vi "Begin.vi"() -> (0 "error out":errorcluster)   [LabVIEW 2018]
doc: "Called before other user functions, this VI can be used to open I/O refnums, load in file data, and do general program initialization. Notice that the <B>error out</B> terminal is simply used for data flow. Wiring it to other structures or subVIs ensures that this VI runs first."
uses:
  <vilib>/Rock Robotics/WPI/DriverStation/WPI_DriverStationRobotMode2.ctl
  <vilib>/Rock Robotics/WPI/Joystick/WPI_JoystickDeviceEnum.ctl
  <vilib>/Rock Robotics/WPI/ThirdParty/REV Robotics/SPARK MAX/Typedef/Spark MAX Status Frames.ctl
  <vilib>/Rock Robotics/WPI/Solenoid/WPI_SolenoidChannel.ctl
  <vilib>/Rock Robotics/WPI/ThirdParty/REV Robotics/SPARK MAX/Typedef/Spark MAX Motor Type.ctl
  <vilib>/Rock Robotics/SystemInterfaces/DIO/FPGA_DIOChannel.ctl
  <vilib>/Rock Robotics/WPI/ThirdParty/REV Robotics/SPARK MAX/Typedef/Spark MAX Idle Mode.ctl
  <vilib>/Rock Robotics/WPI/Solenoid/WPI_SolenoidValue.ctl
  <vilib>/Rock Robotics/WPI/SafetyOutput/WPI_SafetyOutputConfigMenu.ctl
  Odometry/Typedef/Odometry.ctl
  Robot Global Data.vi
  <vilib>/Rock Robotics/Network Tables/NT Write String Array.vi
  <vilib>/Rock Robotics/WPI/Solenoid/WPI_SolenoidOpenDouble.vi
  <vilib>/Rock Robotics/WPI/Counter/WPI_CounterDigitalInputToDigitalSource.vi
  <vilib>/Rock Robotics/WPI/Counter/WPI_CounterOpen Semi Period Mode.vi
  <vilib>/Rock Robotics/WPI/Solenoid/WPI_SolenoidSetEnum.vi
  Asynchronous TDMS Logger/TDMS Logger.lvclass
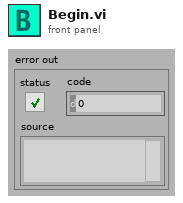
[diagram p1: front panel]
types:
  T1 = typedef "WPI_SafetyOutputConfigMenu.ctl" = enum16{"Enable", "Disable"}
  T2 = typedef "WPI_SolenoidValue.ctl" = enum16{"Off", "On", "Forward", "Reverse"}
  T3 = typedef "WPI_SolenoidChannel.ctl" = enum8{"Solenoid 0", "Solenoid 1", "Solenoid 2", "Solenoid 3", "Solenoid 4", "Solenoid 5", "Solenoid 6", "Solenoid 7", "Invalid"}
  T4 = typedef "FPGA_DIOChannel.ctl" = enum8{"DIO 0", "DIO 1", "DIO 2", "DIO 3", "DIO 4", "DIO 5", "DIO 6", "DIO 7", "DIO 8", "DIO 9", "DIO MXP 0", "DIO MXP 1", "DIO MXP 2", "DIO MXP 3", "DIO MXP 4", "DIO MXP 5", "DIO MXP 6", "DIO MXP 7", "DIO MXP 8", "DIO MXP 9", "DIO MXP 10", "DIO MXP 11", "DIO MXP 12", "DIO MXP 13", "DIO MXP 14", "DIO MXP 15", "SPI Port CS1", "SPI Port CS2", "SPI Port CS3", "SPI Port MISO", "SPI Port MOSI", "Invalid"}
  T5 = typedef "Spark MAX Status Frames.ctl" = enum16{"Status 0", "Status 1", "Status 2"}
  T6 = typedef "Spark MAX Idle Mode.ctl" = enum16{"Coast", "Brake"}
  T7 = typedef "Spark MAX Motor Type.ctl" = enum16{"Brushed", "Brushless"}
  T8 = cluster{"P Gain":dbl, "I Gain":dbl, "D Gain":dbl, "F Gain":dbl, "I Zone":dbl, "Min Output":dbl, "Max Output":dbl}
  T9 = typedef "WPI_JoystickDeviceEnum.ctl" = enum16{"USB 0", "USB 1", "USB 2", "USB 3", "USB 4", "USB 5"}
  T10 = typedef "WPI_DriverStationRobotMode2.ctl" = enum16{"Autonomous Disabled", "Autonomous Enabled", "Teleop Disabled", "Teleop Enabled", "Disconnected", "Finish", "Test Disabled", "Test Enabled", "Emergency Stopped"}
  T11 = typedef "WPI_MotorControlDeviceRef.ctl" = cluster{"DeviceStatus":errorcluster, "Type":T12, "PWM":cluster{"PWM Channel":T13, "DeadBand":T14}, "CAN":cluster{"Device Number":u8, "SetOutput VI Ref":variant, "GetOutput VI Ref":variant, "Enable VI Ref":variant, "Disable VI Ref":variant, "Data":variant}, "Invert":bool, "DIO PWM":cluster{"PWM \"Enable\" Channel":T13, "DIOChannel":T4, "PWM Rate":dbl}}
  T12 = typedef "WPI_MotorControlType.ctl" = enum16{"PWM", "CAN", "DIO PWM"}
  T13 = typedef "FPGA_DIOPWMChannel.ctl" = enum8{"PWM 0", "PWM 1", "PWM 2", "PWM 3", "PWM 4", "PWM 5", "PWM 6", "PWM 7", "PWM 8", "PWM 9", "PWM MXP 0", "PWM MXP 1", "PWM MXP 2", "PWM MXP 3", "PWM MXP 4", "PWM MXP 5", "PWM MXP 6", "PWM MXP 7", "PWM MXP 8", "PWM MXP 9", "Invalid"}
  T14 = typedef "WPI_PWMDeadband.ctl" = cluster{"Name":string, "maxPositivePwm":i32, "minPositivePwm":i32, "centerPwm":i32, "maxNegativePwm":i32, "minNegativePwm":i32, "angularRange":u16}
  T15 = typedef "WPI_DigitalInputDevRef.ctl" = cluster{"DevStatus":errorcluster, "DIO Channel":T4}
  T16 = typedef "FPGA_CounterEncoderSourceConvertionLVSourceType.ctl" = cluster{"DevStatus":errorcluster, "AnalogTriggerMode?":bool, "DigitalMode":cluster{"DIO Channel":T17}, "AnalogTriggerMode":cluster{"AnalogTriggerIndex":T18, "OutputType":T19}}
  T17 = typedef "FPGA_DIODigitalSourceChannel.ctl" = enum8{"DIO 0", "DIO 1", "DIO 2", "DIO 3", "DIO 4", "DIO 5", "DIO 6", "DIO 7", "DIO 8", "DIO 9", "DIO MXP 0", "DIO MXP 1", "DIO MXP 2", "DIO MXP 3", "DIO MXP 4", "DIO MXP 5", "DIO MXP 6", "DIO MXP 7", "DIO MXP 8", "DIO MXP 9", "DIO MXP 10", "DIO MXP 11", "DIO MXP 12", "DIO MXP 13", "DIO MXP 14", "DIO MXP 15", "SPI Port CS1", "SPI Port CS2", "SPI Port CS3", "SPI Port MISO", "SPI Port MOSI", "Disabled"}
  T18 = typedef "FPGA_AnalogTriggerIndex.ctl" = enum8{"Trig 0", "Trig 1", "Trig 2", "Trig 3", "Trig 4", "Trig 5", "Trig 6", "Trig 7", "Invalid"}
  T19 = typedef "FPGA_AnalogTriggerOutType.ctl" = enum16{"InWindow", "TriggerState", "Rising", "Falling"}
  T20 = typedef "WPI_EncoderDevRef.ctl" = cluster{"DevStatus":errorcluster, "EncoderIndex":T21, "CounterIndex":T22, "DistancePerCount":dbl, "Decoding Type":T23}
  T21 = typedef "FPGA_EncoderIdx.ctl" = enum8{"Enc 0", "Enc 1", "Enc 2", "Enc 3", "Enc 4", "Enc 5", "Enc 6", "Enc 7", "Invalid"}
  T22 = typedef "FPGA_CounterCtrSystemIndex.ctl" = enum8{"Ctr 0", "Ctr 1", "Ctr 2", "Ctr 3", "Ctr 4", "Ctr 5", "Ctr 6", "Ctr 7", "Invalid"}
  T23 = typedef "WPI_EncoderType.ctl" = enum16{"1x", "2x", "4x"}
  T24 = typedef "WPI_JoystickDevRef.ctl" = cluster{"Device":T9}
  T25 = typedef "Odometry.ctl" = cluster{"x":dbl, "y":dbl, "theta":dbl, "Left Encoder":dbl, "Right Encoder":dbl, "Late Iterations":i16}
  T26 = typedef "SPARKMAX6Motor.ctl" = cluster{"FrontLeftMaster":T11, "FrontLeftSlave1":T11, "FrontLeftSlave2":T11, "FrontRightMaster":T11, "FrontRightSlave1":T11, "FrontRightSlave2":T11}
  T27 = typedef "WPI_SolenoidDevRef.ctl" = cluster{"DevStatus":errorcluster, "Pneumatics Control Module":u8, "Forward Solenoid Channel":T3, "Reverse Solenoid Channel":T3}
  T28 = typedef "WPI_CounterDevRef.ctl" = cluster{"DevStatus":errorcluster, "CntIndex":T22}
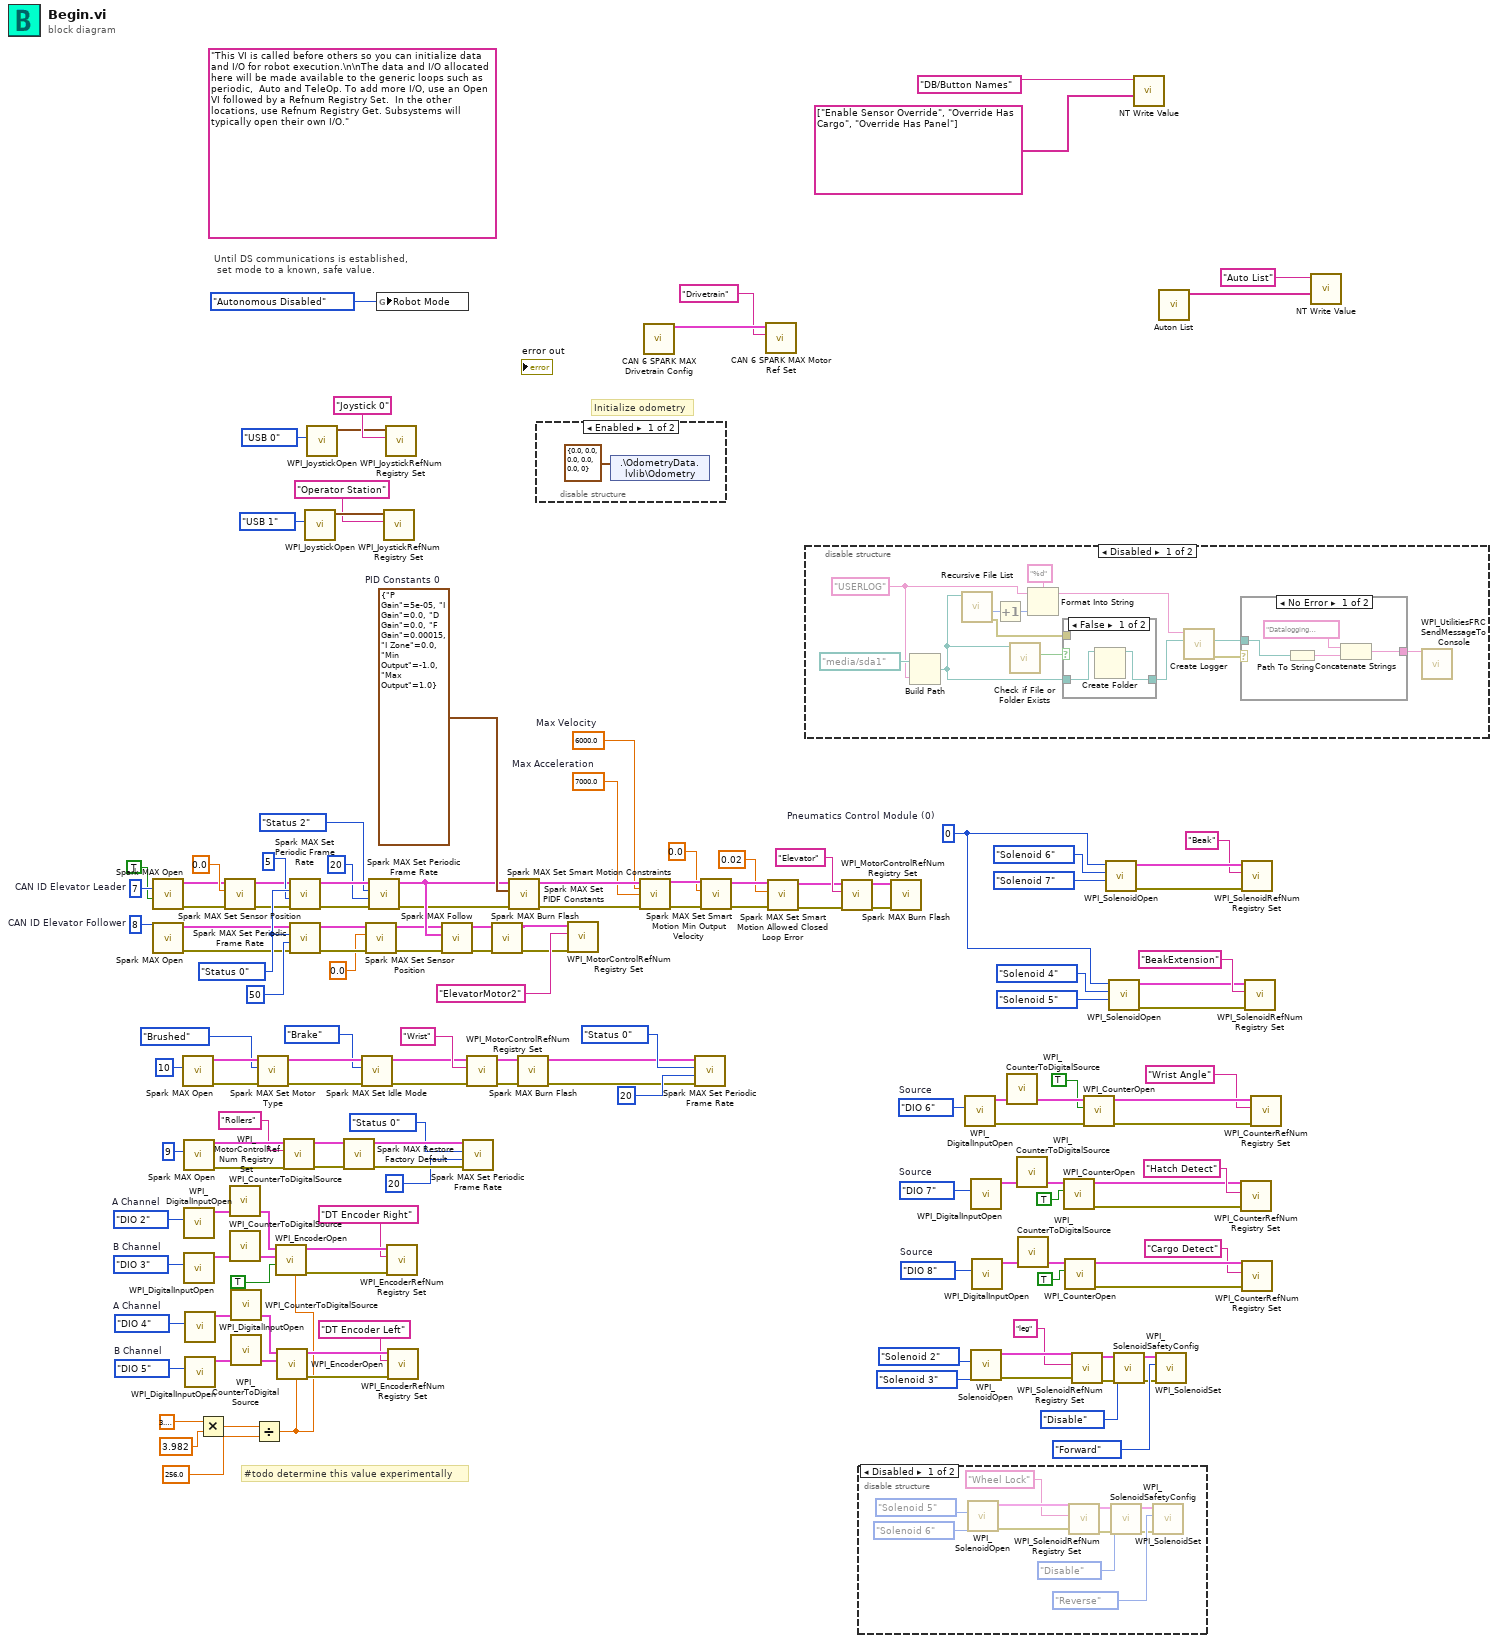
[diagram p0: block diagram]
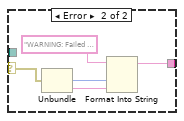
[diagram p5: hidden frame]
diagram:
  w14 = FPGA_DIOChannel."DIO 8"  # Source
  w39 = FPGA_DIOChannel."DIO 5"  # B Channel
  w40 = FPGA_DIOChannel."DIO 4"  # A Channel
  w50 = FPGA_DIOChannel."DIO 3"  # B Channel
  w49 = FPGA_DIOChannel."DIO 2"  # A Channel
  w64 = FPGA_DIOChannel."DIO 7"  # Source
  w80 = 7000.0  # Max Acceleration
  w81 = 6000.0  # Max Velocity
  w94 = FPGA_DIOChannel."DIO 6"  # Source
  w107 = u8 0  # Pneumatics Control Module (0)
  w138 = T8 {"P Gain"=5e-05, "I Gain"=0.0, "D Gain"=0.0, "F Gain"=0.00015, "I Zone"=0.0, "Min Output"=-1.0, "Max Output"=1.0}  # PID Constants 0
  w136 = Spark_MAX_Status_Frames."Status 0" ("Frame")
  w132 = u8 7  # CAN ID Elevator Leader
  w133 = u8 8  # CAN ID Elevator Follower
  (unwired) "This VI is called before others so you can initialize data and I/O for robot execution.\n\nThe data and I/O allocated here will be made available to the generic loops such as periodic,  Auto and TeleOp. To add more I/O, use an Open VI followed by a Refnum Registry Set.  In the other locations, use Refnum Registry Get. Subsystems will typically open their own I/O."
  # "#todo determine this value experimentally"
  # "Initialize odometry"
  # "Until DS communications is established,\n set mode to a known, safe value."
  n1 = call <vilib>:"Spark MAX Open.vi"("Invert"=TRUE, "Device Number"=w132) -> ("error out"=w122:errorcluster, "MotorControlDeviceRef"=w121:T11)  [unwired: 8 in]
  n2 = call <vilib>:"Spark MAX Open.vi"("Device Number"=w133) -> ("error out"=w134:errorcluster, "MotorControlDeviceRef"=w135:T11)  [unwired: 9 in]
  n3 = call <vilib>:"Spark MAX Open.vi"("Device Number"=u8 10) -> ("error out"=w75:errorcluster, "MotorControlDeviceRef"=w99:T11)  [unwired: 9 in]
  n4 = call <vilib>:"Spark MAX Open.vi"("Device Number"=u8 9) -> ("error out"=w68:errorcluster, "MotorControlDeviceRef"=w101:T11)  [unwired: 9 in]
  n5 = call <vilib>:"WPI_DigitalInputOpen.vi"("DIO Channel"=w49) -> ("DigitalInputDevRef"=w46:T15)  [unwired: 1 in, 9 out]
  n6 = call <vilib>:"WPI_DigitalInputOpen.vi"("DIO Channel"=w50) -> ("DigitalInputDevRef"=w47:T15)  [unwired: 1 in, 9 out]
  n7 = call <vilib>:"WPI_DigitalInputOpen.vi"("DIO Channel"=w40) -> ("DigitalInputDevRef"=w43:T15)  [unwired: 1 in, 9 out]
  n8 = call <vilib>:"WPI_DigitalInputOpen.vi"("DIO Channel"=w39) -> ("DigitalInputDevRef"=w42:T15)  [unwired: 1 in, 9 out]
  n9 = Multiply(x=3.141592653589793, y=3.982) -> (x*y=w30:dbl)
  n10 = call <vilib>:"Spark MAX Set Sensor Position.vi"("error in"=w122, "Position"=0.0, "MotorControlDeviceRef"=w121) -> ("error out"=w119:errorcluster, "MotorControlDeviceRef"=w120:T11)  [unwired: 7 in]
  n11 = call-poly <vilib>:"WPI_CounterToDigitalSource.vi"("DigitalInputDevRef"=w46) -> ("Digital Source"=w45:T16)  [unwired: 6 out]
  n12 = call-poly <vilib>:"WPI_CounterToDigitalSource.vi"("DigitalInputDevRef"=w47) -> ("Digital Source"=w48:T16)  [unwired: 6 out]
  n13 = call-poly <vilib>:"WPI_CounterToDigitalSource.vi"("DigitalInputDevRef"=w43) -> ("Digital Source"=w44:T16)  [unwired: 6 out]
  n14 = call-poly <vilib>:"WPI_CounterToDigitalSource.vi"("DigitalInputDevRef"=w42) -> ("Digital Source"=w41:T16)  [unwired: 6 out]
  n15 = Divide(x=w30, y=256.0) -> (x/y=w1:dbl)
  n16 = call <vilib>:"Spark MAX Set Motor Type.vi"("error in (no error)"=w75, "Enum"=Spark_MAX_Motor_Type."Brushed", "MotorControlDevRef"=w99) -> ("error out"=w96:errorcluster, "MotorControlDeviceRef"=w73:T11)  [unwired: 7 in]
  n17 = call <vilib>:"WPI_EncoderOpen.vi"("DistancePerCount"=w1, "Invert Direction (False)"=TRUE, "BSource"=w48, "ASource"=w45) -> ("error out"=w38:errorcluster, "EncoderDevRef"=w35:T20)  [unwired: 4 in, 2 out]
  n18 = call <vilib>:"WPI_EncoderOpen.vi"("DistancePerCount"=w1, "BSource"=w41, "ASource"=w44) -> ("error out"=w37:errorcluster, "EncoderDevRef"=w36:T20)  [unwired: 5 in, 2 out]
  n19 = call <vilib>:"WPI_MotorControlRefNum Registry Set.vi"("error in (no error)"=w68, "refnum name"="Rollers", "MotorControlDevRef"=w101) -> ("error out"=w67:errorcluster, "MotorControlDevRef"=w66:T11)  [unwired: 7 in]
  n20 = call <vilib>:"Spark MAX Set Periodic Frame Rate.vi"("error in"=w119, "Frame rate (ms)"=u16 5, "Frame"=w136, "MotorControlDeviceRef"=w120) -> ("error out"=w131:errorcluster, "MotorControlDeviceRef"=w130:T11)  [unwired: 6 in]
  n21 = call <vilib>:"Spark MAX Set Periodic Frame Rate.vi"("error in"=w134, "Frame rate (ms)"=u16 50, "Frame"=w136, "MotorControlDeviceRef"=w135) -> ("error out"=w54:errorcluster, "MotorControlDeviceRef"=w55:T11)  [unwired: 6 in]
  n22 = call <vilib>:"WPI_JoystickOpen.vi"("JoystickDevice"=WPI_JoystickDeviceEnum."USB 1") -> ("JoystickDevRef"=w145:T24)  [unwired: 10 in]
  n23 = call <vilib>:"WPI_JoystickOpen.vi"("JoystickDevice"=WPI_JoystickDeviceEnum."USB 0") -> ("JoystickDevRef"=w150:T24)  [unwired: 10 in]
  n24 = call <vilib>:"Spark MAX Restore Factory Default.vi"("error in"=w67, "MotorControlDeviceRef"=w66) -> ("error out"=w26:errorcluster, "MotorControlDeviceRef"=w27:T11)  [unwired: 8 in]
  n25 = call <vilib>:"Spark MAX Set Idle Mode.vi"("error in (no error)"=w96, "Idle Mode"=Spark_MAX_Idle_Mode."Brake", "MotorControlDeviceRef in"=w73) -> ("error out"=w74:errorcluster, "MotorControlDeviceRef out"=w72:T11)  [unwired: 7 in]
  n26 = call <vilib>:"Spark MAX Set Sensor Position.vi"("error in"=w54, "Position"=0.0, "MotorControlDeviceRef"=w55) -> ("error out"=w52:errorcluster, "MotorControlDeviceRef"=w53:T11)  [unwired: 7 in]
  n27 = call <vilib>:"Spark MAX Set Periodic Frame Rate.vi"("error in"=w131, "Frame rate (ms)"=u16 20, "Frame"=Spark_MAX_Status_Frames."Status 2", "MotorControlDeviceRef"=w130) -> ("error out"=w127:errorcluster, "MotorControlDeviceRef"=w129:T11)  [unwired: 6 in]
  n28 = global write "Robot Global Data.vi" "Robot Mode"(WPI_DriverStationRobotMode2."Autonomous Disabled" ("Robot Mode")) -> ()
  n29 = call <vilib>:"WPI_JoystickRefNum Registry Set.vi"("refnum name"="Operator Station", "JoystickDevRef"=w145) -> ()  [unwired: 8 in, 2 out]
  n30 = call <vilib>:"WPI_JoystickRefNum Registry Set.vi"("refnum name"="Joystick 0", "JoystickDevRef"=w150) -> ()  [unwired: 8 in, 2 out]
  n31 = call <vilib>:"WPI_EncoderRefNum Registry Set.vi"("error in (no error)"=w38, "refnum name"="DT Encoder Right", "EncoderDevRef"=w35) -> ()  [unwired: 7 in, 2 out]
  n32 = call <vilib>:"WPI_EncoderRefNum Registry Set.vi"("error in (no error)"=w37, "refnum name"="DT Encoder Left", "EncoderDevRef"=w36) -> ()  [unwired: 7 in, 2 out]
  n33 = call <vilib>:"Spark MAX Follow.vi"("error in (no error)"=w52, "Master Controller"=w129, "MotorControlDeviceRef"=w53) -> ("error out"=w105:errorcluster, "MotorControlDeviceRef"=w104:T11)  [unwired: 7 in]
  n34 = call <vilib>:"Spark MAX Set Periodic Frame Rate.vi"("error in"=w26, "Frame rate (ms)"=u16 20, "Frame"=Spark_MAX_Status_Frames."Status 0", "MotorControlDeviceRef"=w27) -> ()  [unwired: 6 in, 2 out]
  n35 = call <vilib>:"WPI_MotorControlRefNum Registry Set.vi"("error in (no error)"=w74, "refnum name"="Wrist", "MotorControlDevRef"=w72) -> ("error out"=w70:errorcluster, "MotorControlDevRef"=w69:T11)  [unwired: 7 in]
  n36 = call <vilib>:"Spark MAX Burn Flash.vi"("error in"=w105, "MotorControlDeviceRef"=w104) -> ("error out"=w57:errorcluster, "MotorControlDeviceRef"=w56:T11)  [unwired: 8 in]
  n37 = call <vilib>:"Spark MAX Set PIDF Constants.vi"("error in"=w127, "PID Constants"=w138, "MotorControlDeviceRef"=w129) -> ("error out"=w125:errorcluster, "MotorControlDeviceRef"=w124:T11)  [unwired: 7 in]
  n38 = call <vilib>:"Spark MAX Burn Flash.vi"("error in"=w70, "MotorControlDeviceRef"=w69) -> ("error out"=w20:errorcluster, "MotorControlDeviceRef"=w21:T11)  [unwired: 8 in]
  n39 = disable-structure shown="Enabled" {
    frame Enabled {
      n40 = shared-variable ".\\OdometryData.lvlib\\Odometry"(T25 {"x"=0.0, "y"=0.0, "theta"=0.0, "Left Encoder"=0.0, "Right Encoder"=0.0, "Late Iterations"=0} ("Odometry")) -> ()  [unwired: 1 in, 1 out]
    }
    frame Disabled {
    }
  }
  n41 = call <vilib>:"WPI_MotorControlRefNum Registry Set.vi"("error in (no error)"=w57, "refnum name"="ElevatorMotor2", "MotorControlDevRef"=w56) -> ()  [unwired: 7 in, 2 out]
  n42 = call <vilib>:"Spark MAX Set Smart Motion Constraints.vi"("MotorControlDeviceRef"=w124, "Max Velocity"=w81, "Max Acceleration"=w80, "error in"=w125) -> ("MotorControlDeviceRef"=w86:T11, "error out"=w87:errorcluster)  [unwired: 10 in]
  n43 = call "CAN 6 SPARK MAX Drivetrain Config.vi"() -> ("SPARK MAX Ref"=w141:T26)  [unwired: 19 in]
  n44 = call <vilib>:"Spark MAX Set Periodic Frame Rate.vi"("error in"=w20, "Frame rate (ms)"=u16 20, "Frame"=Spark_MAX_Status_Frames."Status 0", "MotorControlDeviceRef"=w21) -> ()  [unwired: 6 in, 2 out]
  n45 = call <vilib>:"Spark MAX Set Smart Motion Min Output Velocity.vi"("error in"=w87, "Minimum Velocity Output"=0.0, "MotorControlDeviceRef"=w86) -> ("error out"=w85:errorcluster, "MotorControlDeviceRef"=w84:T11)  [unwired: 7 in]
  n46 = call "CAN 6 SPARK MAX Motor Ref Set.vi"("refnum name"="Drivetrain", "TalonSRX6MotorRef in"=w141) -> ()  [unwired: 8 in, 2 out]
  n47 = call <vilib>:"Spark MAX Set Smart Motion Allowed Closed Loop Error.vi"("error in"=w85, "Allowed Closed Loop Error"=0.02, "MotorControlDeviceRef"=w84) -> ("error out"=w83:errorcluster, "MotorControlDeviceRef"=w82:T11)  [unwired: 7 in]
  n48 = disable-structure shown="Disabled" {
    frame Disabled {
      w161 = "USERLOG" ("Base File Name")
      n49 = Build Path(base path=path "/media/sda1", name or relative path=w161) -> (appended path=w163:path)
      n50 = call <vilib>:"Recursive File List.vi"("Folder Path"=w163) -> ("error out"=w158:errorcluster, "Number of Files"=w162:i32)  [unwired: 6 in, 3 out]
      n51 = Increment(x=w162) -> (x+1=w160:i32)
      n52 = call <vilib>:"Check if File or Folder Exists.vi"("path"=w163) -> ("file or folder exists?"=w164:bool)  [unwired: 8 in, 2 out]
      n53 = Format Into String(format string="%d", initial string=w161, w160) -> (resulting string=w157:string)  [unwired: 1 in, 1 out]
      n54 = case shown="False" w164 {
        tunnel: w163 -> [w168 w169]
        tunnel: [w167 w169] -> w154
        tunnel: w158 -> [_ _]
        frame False {
          n55 = Create Folder(path (use dialog)=w168) -> (created path=w167:path)  [unwired: 2 in, 2 out]
        }
        frame True {
        }
      }
      n56 = call "Create Logger.vi"("Base Folder"=w154, "Base File Name"=w157) -> ("Error Out"=w155:errorcluster, "Final Path"=w156:path)  [unwired: 7 in, 1 out]
      n57 = case shown="No Error" w155 {
        selector: w155 -> [_ w177]
        tunnel: w156 -> [w173 _]
        tunnel: [w170 w174] -> w166
        frame No Error {
          n58 = Path To String(path=w173) -> (string=w172:string)
          n59 = Concatenate Strings("Datalogging Initialized to: " ("string"), w172) -> (w170:string)
        }
        frame Error {
          n60 = Unbundle(w177) -> ("code"=w176:i32, "source"=w175:string)  [unwired: 1 out]
          n61 = Format Into String(initial string="WARNING: Failed to initialize datalogger! " ("string"), w176, w175) -> (resulting string=w174:string)  [unwired: 2 in, 1 out]
        }
      }
      n62 = call <vilib>:"WPI_UtilitiesFRC SendMessageToConsole.vi"("Message"=w166) -> ()  [unwired: 14 in, 1 out]
    }
    frame Enabled {
    }
  }
  n63 = call <vilib>:"WPI_MotorControlRefNum Registry Set.vi"("error in (no error)"=w83, "refnum name"="Elevator", "MotorControlDevRef"=w82) -> ("error out"=w76:errorcluster, "MotorControlDevRef"=w77:T11)  [unwired: 7 in]
  n64 = disable-structure shown="Disabled" {
    frame Disabled {
      n65 = call-poly <vilib>:"WPI_SolenoidOpen.vi"("Reverse Solenoid Channel"=WPI_SolenoidChannel."Solenoid 6", "Forward Solenoid Channel"=WPI_SolenoidChannel."Solenoid 5" ("Solenoid Channel")) -> ("error out"=w187:errorcluster, "SolenoidDevRef"=w189:T27)  [unwired: 8 in]
      n66 = call <vilib>:"WPI_SolenoidRefNum Registry Set.vi"("error in (no error)"=w187, "refnum name"="Wheel Lock", "SolenoidDevRef"=w189) -> ("error out"=w182:errorcluster, "SolenoidDevRef"=w183:T27)  [unwired: 7 in]
      n67 = call <vilib>:"WPI_SolenoidSafetyConfig.vi"("error in (no error)"=w182, "mode"=WPI_SafetyOutputConfigMenu."Disable", "SolenoidDevRef"=w183) -> ("error out"=w180:errorcluster, "SolenoidDevRef"=w181:T27)  [unwired: 7 in]
      n68 = call-poly <vilib>:"WPI_SolenoidSet.vi"("error in (no error)"=w180, "Value"=WPI_SolenoidValue."Reverse", "SolenoidDevRef"=w181) -> ()  [unwired: 7 in, 2 out]
    }
    frame Enabled {
    }
  }
  n69 = call <vilib>:"Spark MAX Burn Flash.vi"("error in"=w76, "MotorControlDeviceRef"=w77) -> ()  [unwired: 8 in, 2 out]
  n70 = call <vilib>:"WPI_DigitalInputOpen.vi"("DIO Channel"=w94) -> ("error out"=w92:errorcluster, "DigitalInputDevRef"=w93:T15)  [unwired: 1 in, 8 out]
  n71 = call <vilib>:"WPI_DigitalInputOpen.vi"("DIO Channel"=w64) -> ("DigitalInputDevRef"=w63:T15)  [unwired: 1 in, 9 out]
  n72 = call-poly <vilib>:"WPI_SolenoidOpen.vi"("Reverse Solenoid Channel"=WPI_SolenoidChannel."Solenoid 3", "Forward Solenoid Channel"=WPI_SolenoidChannel."Solenoid 2" ("Solenoid Channel")) -> ("error out"=w10:errorcluster, "SolenoidDevRef"=w12:T27)  [unwired: 8 in]
  n73 = call <vilib>:"WPI_DigitalInputOpen.vi"("DIO Channel"=w14) -> ("DigitalInputDevRef"=w15:T15)  [unwired: 1 in, 9 out]
  n74 = call-poly <vilib>:"WPI_CounterToDigitalSource.vi"("DigitalInputDevRef"=w93) -> ("Digital Source"=w95:T16)  [unwired: 6 out]
  n75 = call-poly <vilib>:"WPI_CounterToDigitalSource.vi"("DigitalInputDevRef"=w63) -> ("Digital Source"=w65:T16)  [unwired: 6 out]
  n76 = call-poly <vilib>:"WPI_CounterToDigitalSource.vi"("DigitalInputDevRef"=w15) -> ("Digital Source"=w13:T16)  [unwired: 6 out]
  n77 = call-poly <vilib>:"WPI_CounterOpen.vi"("High Pulse (T)"=TRUE, "Source"=w65) -> ("error out"=w59:errorcluster, "CounterDevRef"=w60:T28)  [unwired: 3 in, 5 out]
  n78 = call-poly <vilib>:"WPI_CounterOpen.vi"("High Pulse (T)"=TRUE, "Source"=w13) -> ("error out"=w19:errorcluster, "CounterDevRef"=w18:T28)  [unwired: 3 in, 5 out]
  n79 = call <vilib>:"WPI_SolenoidRefNum Registry Set.vi"("error in (no error)"=w10, "refnum name"="leg", "SolenoidDevRef"=w12) -> ("error out"=w5:errorcluster, "SolenoidDevRef"=w6:T27)  [unwired: 7 in]
  n80 = call-poly <vilib>:"WPI_CounterOpen.vi"("error in (no error)"=w92, "High Pulse (T)"=TRUE, "Source"=w95) -> ("error out"=w90:errorcluster, "CounterDevRef"=w91:T28)  [unwired: 2 in, 5 out]
  n81 = call-poly <vilib>:"WPI_SolenoidOpen.vi"("Reverse Solenoid Channel"=WPI_SolenoidChannel."Solenoid 7", "Forward Solenoid Channel"=WPI_SolenoidChannel."Solenoid 6", "Pneumatics Control Module (0)"=w107) -> ("error out"=w116:errorcluster, "SolenoidDevRef"=w117:T27)  [unwired: 7 in]
  n82 = call-poly <vilib>:"WPI_SolenoidOpen.vi"("Reverse Solenoid Channel"=WPI_SolenoidChannel."Solenoid 5", "Forward Solenoid Channel"=WPI_SolenoidChannel."Solenoid 4", "Pneumatics Control Module (0)"=w107) -> ("error out"=w109:errorcluster, "SolenoidDevRef"=w108:T27)  [unwired: 7 in]
  n83 = call <vilib>:"WPI_SolenoidSafetyConfig.vi"("error in (no error)"=w5, "mode"=WPI_SafetyOutputConfigMenu."Disable", "SolenoidDevRef"=w6) -> ("error out"=w3:errorcluster, "SolenoidDevRef"=w4:T27)  [unwired: 7 in]
  n84 = call-poly <vilib>:"NT Write Value.vi"("String Array"=string[] ["Enable Sensor Override", "Override Has Cargo", "Override Has Panel"], "Name"="DB/Button Names") -> ()  [unwired: 9 in, 1 out]
  n85 = call-poly <vilib>:"WPI_SolenoidSet.vi"("error in (no error)"=w3, "Value"=WPI_SolenoidValue."Forward", "SolenoidDevRef"=w4) -> ()  [unwired: 7 in, 2 out]
  n86 = call "Auton List.vi"() -> ("String Array"=w142:string[])  [unwired: 11 in]
  n87 = call <vilib>:"WPI_CounterRefNum Registry Set.vi"("error in (no error)"=w59, "refnum name"="Hatch Detect", "CounterDevRef"=w60) -> ()  [unwired: 7 in, 2 out]
  n88 = call <vilib>:"WPI_SolenoidRefNum Registry Set.vi"("error in (no error)"=w116, "refnum name"="Beak", "SolenoidDevRef"=w117) -> ()  [unwired: 7 in, 2 out]
  n89 = call <vilib>:"WPI_CounterRefNum Registry Set.vi"("error in (no error)"=w19, "refnum name"="Cargo Detect", "CounterDevRef"=w18) -> ()  [unwired: 7 in, 2 out]
  n90 = call <vilib>:"WPI_SolenoidRefNum Registry Set.vi"("error in (no error)"=w109, "refnum name"="BeakExtension", "SolenoidDevRef"=w108) -> ()  [unwired: 7 in, 2 out]
  n91 = call <vilib>:"WPI_CounterRefNum Registry Set.vi"("error in (no error)"=w90, "refnum name"="Wrist Angle", "CounterDevRef"=w91) -> ()  [unwired: 7 in, 2 out]
  n92 = call-poly <vilib>:"NT Write Value.vi"("String Array"=w142, "Name"="Auto List") -> ()  [unwired: 9 in, 1 out]
